vi "Create_Csv_Data.vi"(6 "N":i32, 9 "Head":T1={"File"=[refnum], "Idx"=[], "dT"=0.5, "Hd"=4096, "Rd"=14, "Start"=[timestamp(3519879471 s since 1904-01-01)], "Trig"=[timestamp(3519879472 s since 1904-01-01)], "Stop"=[timestamp(3519940623 s since 1904-01-01)], "FirstPos"=[], "Count"=[120609], "Color"=[27836, 4765252, 11010216, 14712848], "Label"=["CH1", "CH2", "CH3", "CH4"], "INP"=["CH1", "CH2", "CH3", "CH4"], "H"=[5.0, 5.0, 5.0, 5.0], "L"=[-5.0, -5.0, -5.0, -5.0], "Fmt"=["%.;%+0.3f V", "%.;%+0.3f V", "%.;%+0.3f V", "%.;%+0.3f V"], "Unit"=["", "", "", ""], "SEL"=[0, 1, 2, 3], "Byte"=[-2, -2, -2, -2], "Pos"=[], "Bit"=[], "Flg"=[], "Gain"=[0.01, 0.01, 0.01, 0.01], "Offset"=[0.0, 0.0, 0.0, 0.0], "CH"=[0, 1, 2, 3], "Opt"={"Mode"=0, "TUNIT"=enum."CELS"}, "TYPE"=enum."GBD", "Comp"=[], "Temp"=[]} {"FirstPos" format="%<%x %.3X>T"; "Stop" format="%<%x %.3X>T"; "Trig" format="%<%x %.3X>T"; "Start" format="%<%x %.3X>T"}, 10 "Bin":string, 11 "Reference":refnum<k24>) -> (1 "CSV":string[](array[string]), 2 "Array":dbl[][](array[numeric]), 4 "Cnt":i32)   [LabVIEW 2017]
uses:
  Amp_Param.ctl
  D:/src/LabVIEW/GL860/JP/LabView VI/64bitdll/GLSampleProgram.dll
  64bitdll/GLSampleProgram.dll
panel:
  # "ALL"
  # "GBD"
  # "CSV"
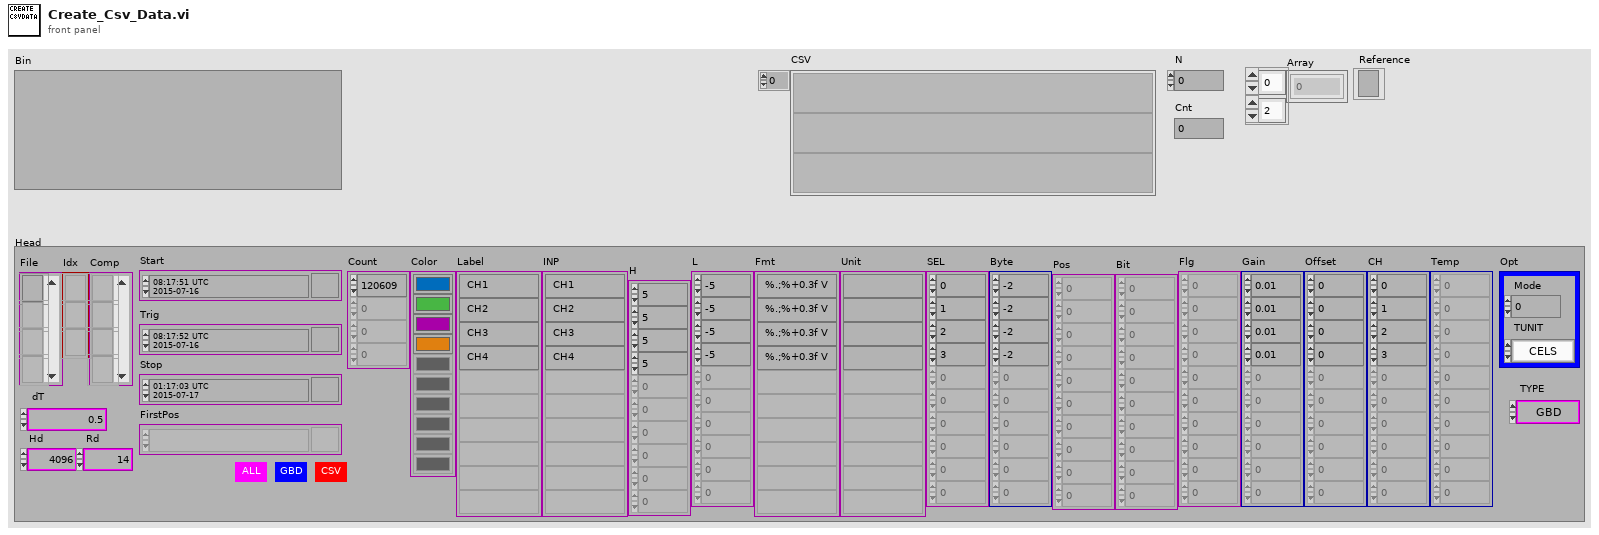
[diagram p1: front panel]
types:
  T1 = typedef "Amp_Param.ctl" = cluster{"File":refnum<file>[], "Idx":refnum<file>[], "dT":dbl, "Hd":i32, "Rd":i32, "Start":timestamp[], "Trig":timestamp[], "Stop":timestamp[], "FirstPos":timestamp[], "Count":i64[], "Color":u32[], "Label":string[], "INP":string[], "H":dbl[], "L":dbl[], "Fmt":string[], "Unit":string[], "SEL":i32[], "Byte":i32[], "Pos":i32[], "Bit":i32[], "Flg":i32[], "Gain":dbl[], "Offset":dbl[], "CH":i32[], "Opt":cluster{"Mode":i32, "TUNIT":enum16{"CELS", "FAHR"}}, "TYPE":enum16{"GBD", "CSV"}, "Comp":refnum<file>[], "Temp":i32[]}
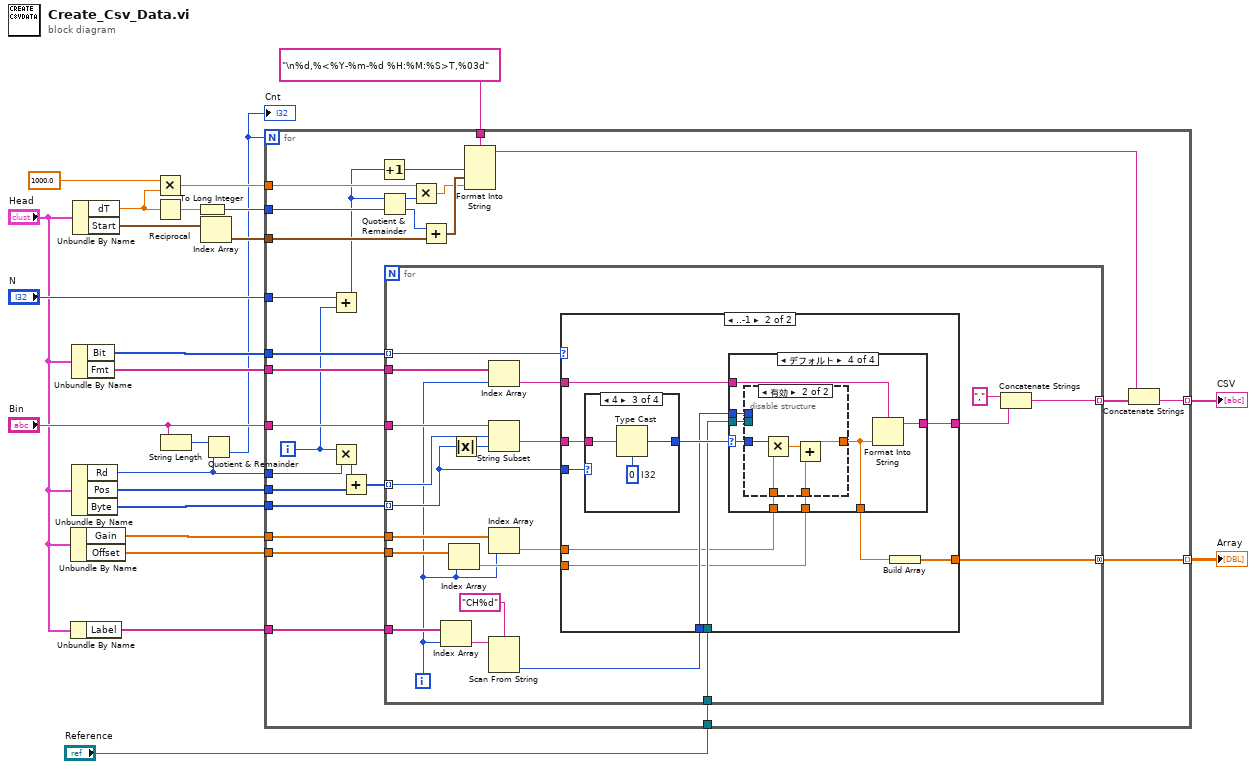
[diagram p0: block diagram]
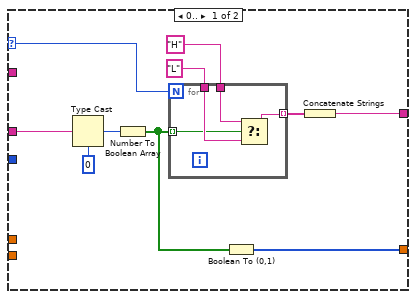
[diagram p2: hidden frame]
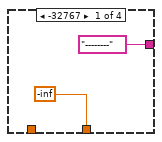
[diagram p3: hidden frame]
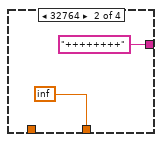
[diagram p4: hidden frame]
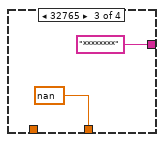
[diagram p5: hidden frame]
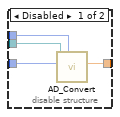
[diagram p6: hidden frame]
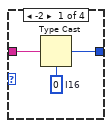
[diagram p7: hidden frame]
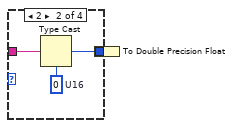
[diagram p8: hidden frame]
diagram:
  n1 = Unbundle By Name("Head") -> ("Gain"=w2:dbl[], "Offset"=w1:dbl[])
  n2 = Unbundle By Name("Head") -> ("Label"=w6:string[])
  n3 = Unbundle By Name("Head") -> ("Bit"=w22:i32[], "Fmt"=w17:string[])
  n4 = Unbundle By Name("Head") -> ("Rd"=w18:i32, "Pos"=w24:i32[], "Byte"=w23:i32[])
  n5 = Unbundle By Name("Head") -> ("dT"=w10:dbl, "Start"=w13:timestamp[])
  n6 = Multiply(x=1000.0, y=w10) -> (x*y=w8:dbl)
  n7 = Reciprocal(x=w10) -> (1/x=w16:dbl)
  n8 = String Length(string="Bin") -> (length=w19:i32)
  n9 = To Long Integer(number=w16) -> (32bit integer=w14:i32)
  n10 = Index Array(array=w13) -> (element=w12:timestamp)  [unwired: 1 in]
  n11 = Quotient & Remainder(x=w19, y=w18) -> (floor(x/y)=w5:i32)  [unwired: 1 out]
  "Cnt" <- w5
  n12 = for {
    N: w5 -> [_]
    tunnel: "Bin" -> [w52]
    tunnel: w24 -> [w42]
    tunnel: w23 -> [w51]
    tunnel: w18 -> [w50]
    tunnel: [w48] -> w21 mode=indexing
    tunnel: w22 -> [w47]
    tunnel: w17 -> [w46]
    tunnel: "N" -> [w45]
    tunnel: w14 -> [w40]
    tunnel: w12 -> [w37]
    tunnel: "\n%d,%<%Y-%m-%d %H:%M:%S>T,%03d" -> [w35]
    tunnel: w8 -> [w32]
    tunnel: [w30] -> w7 mode=indexing
    tunnel: w6 -> [w29]
    tunnel: "Reference" -> [w27]
    tunnel: w2 -> [w26]
    tunnel: w1 -> [w25]
    i -> [w44]
    n13 = Add(x=w45, y=w44) -> (x+y=w31:i32)
    n14 = Multiply(x=w44, y=w50) -> (x*y=w43:i32)
    n15 = Add(x=w43, y=w42) -> (x+y=w41:i32[])
    n16 = Increment(x=w31) -> (x+1=w28:i32)
    n17 = Quotient & Remainder(x=w31, y=w40) -> (x-y*floor(x/y)=w39:i32, floor(x/y)=w36:i32)
    n18 = for {
      tunnel: w51 -> [w72] mode=indexing
      tunnel: w52 -> [w74]
      tunnel: [w73] -> w49 mode=indexing
      tunnel: w47 -> [w71] mode=indexing
      tunnel: w46 -> [w69]
      tunnel: w41 -> [w67] mode=indexing
      tunnel: [w66] -> w30 mode=concatenating
      tunnel: w29 -> [w65]
      tunnel: w27 -> [w59]
      tunnel: w26 -> [w58]
      tunnel: w25 -> [w57]
      i -> [w54]
      n19 = Index Array(array=w65, index=w54) -> (element=w61:string)
      n20 = Index Array(array=w57, index=w54) -> (element=w55:dbl)
      n21 = Absolute Value(x=w72) -> (abs(x)=w70:i32)
      n22 = Index Array(array=w69, index=w54) -> (element=w68:string)
      n23 = String Subset(string=w74, offset (0)=w67, length (rest)=w70) -> (substring=w62:string)
      n24 = Index Array(array=w58, index=w54) -> (element=w56:dbl)
      n25 = Scan From String(format string="CH%d", input string=w61) -> (output 1=w53:i32)  [unwired: 3 in, 3 out]
      n26 = case shown="..-1" w71 {
        selector: w71 -> [w77 _]
        tunnel: w62 -> [w80 w99]
        tunnel: [w81 w97] -> w63
        tunnel: w72 -> [_ w98]
        tunnel: w68 -> [_ w96]
        tunnel: [w75 w94] -> w66
        tunnel: w53 -> [_ w92]
        tunnel: w59 -> [_ w91]
        tunnel: w56 -> [_ w90]
        tunnel: w55 -> [_ w89]
        frame 0.. {
          n27 = Type Cast(type=u16 0, x=w80) -> (*(type *) &x=w79:u16)
          n28 = Number To Boolean Array(number=w79) -> (Boolean array=w76:bool[])
          n29 = for {
            N: w77 -> [_]
            tunnel: w76 -> [w85] mode=indexing
            tunnel: "H" -> [w88]
            tunnel: "L" -> [w87]
            tunnel: [w86] -> w82 mode=indexing
            n30 = Select(t=w88, s=w85, f=w87) -> (s? t:f=w86:string)
          }
          n31 = Boolean To (0,1)(Boolean=w76) -> (0, 1=w75:i16[])
          n32 = Concatenate Strings(w82) -> (w81:string)
        }
        frame ..-1 {
          n33 = case shown="4" w98 {
            tunnel: w99 -> [w124 w126 w130 _]
            tunnel: [w123 _ w129 _] -> w93
            frame -2 {
              w125 = i16 0  # I16
              n34 = Type Cast(type=w125, x=w124) -> (*(type *) &x=w123:i16)
            }
            frame 2 {
              w127 = u16 0  # U16
              n35 = Type Cast(type=w127, x=w126) -> (*(type *) &x=w128:u16)
              n36 = To Double Precision Float(number=w128) -> ()  [unwired: 1 out]
            }
            frame 4 {
              w131 = 0  # I32
              n37 = Type Cast(type=w131, x=w130) -> (*(type *) &x=w129:i32)
            }
            frame Default {
            }
          }
          n38 = case shown="デフォルト" w93 {
            selector: w93 -> [_ _ _ w110]
            tunnel: ["--------" "++++++++" "********" w113] -> w97
            tunnel: w96 -> [_ _ _ w112]
            tunnel: [-inf inf nan w111] -> w95
            tunnel: w92 -> [_ _ _ w109]
            tunnel: w91 -> [_ _ _ w108]
            tunnel: w90 -> [_ _ _ w107]
            tunnel: w89 -> [_ _ _ w106]
            frame -32767 {
            }
            frame 32764 {
            }
            frame 32765 {
            }
            frame Default {
              n39 = disable-structure shown="有効" {
                disable-tunnel: [w117 w118] -> w111
                disable-tunnel: w110 -> [w116 w122]
                disable-tunnel: w109 -> [w115 _]
                disable-tunnel: w108 -> [w114 _]
                disable-tunnel: w107 -> [_ w121]
                disable-tunnel: w106 -> [_ w119]
                frame Disabled {
                  n40 = call "AD_Convert.vi"("CH"=w115, "Data"=w116, "Reference.In"=w114) -> ("AD"=w117:dbl)  [unwired: 6 in, 2 out]
                }
                frame Enabled {
                  n41 = Multiply(x=w122, y=w121) -> (x*y=w120:dbl)
                  n42 = Add(x=w120, y=w119) -> (x+y=w118:dbl)
                }
              }
              n43 = Format Into String(format string=w112, w111) -> (resulting string=w113:string)  [unwired: 2 in, 1 out]
            }
          }
          n44 = Build Array(w95) -> (w94:dbl[])
        }
      }
      n45 = Concatenate Strings(",", w63) -> (w73:string)
    }
    n46 = Multiply(x=w32, y=w39) -> (x*y=w33:dbl)
    n47 = Add(x=w36, y=w37) -> (x+y=w38:timestamp)
    n48 = Format Into String(format string=w35, w28, w38, w33) -> (resulting string=w34:string)  [unwired: 2 in, 1 out]
    n49 = Concatenate Strings(w34, w49) -> (w48:string)
  }
  "CSV" <- w21
  "Array" <- w7
